vi "Test TCRS Update Ramp Rate While Running.vi"(8 "error in (no error)":errorcluster, 11 "Thermal Chamber Response Simlator Test In":refnum<class "Thermal Chamber Response Simlator Test.lvclass">) -> (0 "error out":errorcluster, 3 "Thermal Chamber Response Simlator Test Out":refnum<class "Thermal Chamber Response Simlator Test.lvclass">)   [LabVIEW 2020, in "Thermal Chamber Response Simlator Test.lvclass"]
uses:
  Thermal Chamber Response Simlator Test.lvclass
  C:/Program Files (x86)/National Instruments/LabVIEW 2020/vi.lib/Astemes/LUnit/Test Case.lvclass
  Thermal Chamber Response Simlator/Thermal Chamber Response Simlator.lvclass
  Thermal Chamber Response Simlator/Thermal Chamber Response Simlator.lvclass/Thermal Chamber Response Simlator.ctl
  <vilib>/Astemes/LUnit/Test Case.lvclass/Test Case.ctl
  5d883c7a-c249-4dce-989b-a0d0f0b4e95d.vi
  <vilib>/Astemes/LUnit/Core/LUnit Test Case/Private/Append Pass Result.vi
  <vilib>/Astemes/LUnit/Core/LUnit Test Case/Private/Append Fail Result.vi
  5d883c7a-c249-4dce-989b-a0d0f0b4e95d.vi/9c5d11cd-9439-4240-a1ee-d9baace9c924.vi
  <vilib>/Astemes/LUnit/Core/LUnit Test Case/Private/Run In UI.vi
  <vilib>/Utility/error.llb/Clear Errors.vi
  Thermal Chamber Response Simlator/Private/Get Current Time if Not Set.vi
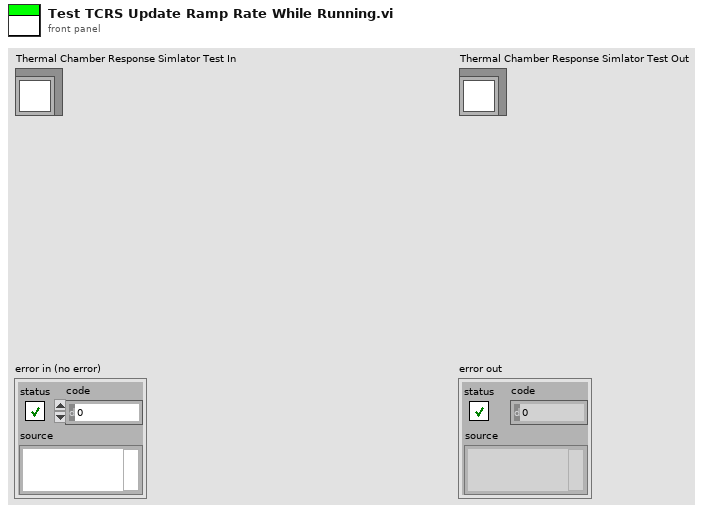
[diagram p1: front panel]
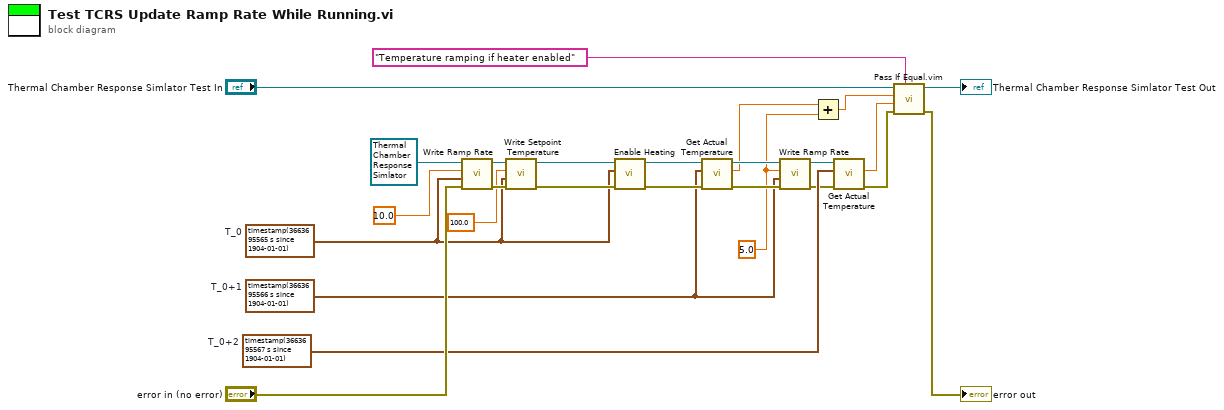
[diagram p0: block diagram]
diagram:
  w8 = timestamp(3663695567 s since 1904-01-01)  # T_0+2
  w2 = 5.0 ("Ramp Rate [degC/s]")
  w9 = timestamp(3663695566 s since 1904-01-01)  # T_0+1
  w11 = timestamp(3663695565 s since 1904-01-01)  # T_0
  n1 = call "Write Ramp Rate.vi"("error in (no error)"="error in (no error)", "Time Stamp"=w11, "Ramp Rate [degC/s]"=10.0, "Thermal Chamber Response Simlator In"=refnum<class "Thermal Chamber Response Simlator.lvclass"> refnum ("Thermal Chamber Response Simlator.lvclass")) -> ("error out"=w24:errorcluster, "Thermal Chamber Response Simlator Out"=w14:refnum<class "Thermal Chamber Response Simlator.lvclass">)  [unwired: 6 in]
  n2 = call "Write Setpoint Temperature.vi"("error in (no error)"=w24, "Update Time"=w11, "Setpoint Temperature [degC]"=100.0, "Thermal Chamber Response Simlator In"=w14) -> ("error out"=w15:errorcluster, "Thermal Chamber Response Simlator Out"=w13:refnum<class "Thermal Chamber Response Simlator.lvclass">)  [unwired: 6 in]
  n3 = call "Enable Heating.vi"("error in (no error)"=w15, "Start Time"=w11, "Thermal Chamber Response Simlator In"=w13) -> ("error out"=w18:errorcluster, "Thermal Chamber Response Simlator Out"=w17:refnum<class "Thermal Chamber Response Simlator.lvclass">)  [unwired: 7 in]
  n4 = call "Get Actual Temperature.vi"("error in (no error)"=w18, "Time Stamp"=w9, "Thermal Chamber Response Simlator In"=w17) -> ("error out"=w22:errorcluster, "Actual Temperature [degC]"=w3:dbl, "Thermal Chamber Response Simlator Out"=w10:refnum<class "Thermal Chamber Response Simlator.lvclass">)  [unwired: 6 in]
  n5 = call "Write Ramp Rate.vi"("error in (no error)"=w22, "Time Stamp"=w9, "Ramp Rate [degC/s]"=w2, "Thermal Chamber Response Simlator In"=w10) -> ("error out"=w6:errorcluster, "Thermal Chamber Response Simlator Out"=w7:refnum<class "Thermal Chamber Response Simlator.lvclass">)  [unwired: 6 in]
  n6 = Add(x=w3, y=w2) -> (x+y=w1:dbl)
  n7 = call "Get Actual Temperature.vi"("error in (no error)"=w6, "Time Stamp"=w8, "Thermal Chamber Response Simlator In"=w7) -> ("error out"=w5:errorcluster, "Actual Temperature [degC]"=w4:dbl)  [unwired: 6 in, 1 out]
  n8 = call "Pass If Equal.vim"("Description"="Temperature ramping if heater enabled", "error in (no error)"=w5, "Actual"=w4, "Expected"=w1, "LUnit Test Case In"="Thermal Chamber Response Simlator Test In") -> ("error out"=→"error out":errorcluster, "LUnit Test Case Out"=→"Thermal Chamber Response Simlator Test Out":refnum<class "Thermal Chamber Response Simlator Test.lvclass">)  [unwired: 5 in]
